vi "Key Event to Bytes.vi"(8 "error in (no error)":errorcluster, 10 "Key Event Data":T1, 11 "Terminal in":refnum<class "Terminal.lvclass">) -> (0 "error out":errorcluster, 2 "String":string, 3 "Terminal out":refnum<class "Terminal.lvclass">)   [LabVIEW 2020, in "Terminal.lvlib" / "Terminal.lvclass"]
uses:
  Terminal.lvclass
  Key Event Data.ctl
  <vilib>/event_ctls.llb/eventvkey.ctl
  Terminal.lvclass/Terminal.ctl
  Terminal.lvlib
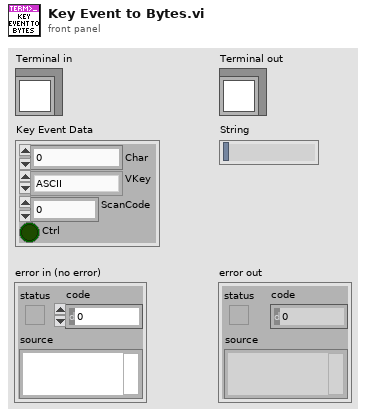
[diagram p1: front panel]
types:
  T1 = typedef "Terminal.lvlib/Key Event Data.ctl" = cluster{"Char":i16, "VKey":T2, "ScanCode":i16, "Ctrl":bool}
  T2 = typedef "eventvkey.ctl" = enum16{"ASCII", "Enter", "Return", "Shift", "Ctrl", "Alt", "Cmd", "Opt", "Caps", "NumLock", "Clear", "Break", "Up", "Down", "Left", "Right", "Insert", "Delete", "Home", "End", "PageUp", "PageDown", "Escape", "Help", "Pause", "ScrollLock", "F1", "F2", "F3", "F4", "F5", "F6", "F7", "F8", "F9", "F10", "F11", "F12", "F13", "F14", "F15", "F16", "F17", "F18", "F19", "F20", "F21", "F22", "F23", "F24", "Play", "VolumeUp", "VolumeDown", "Mute", "Two Byte Char"}
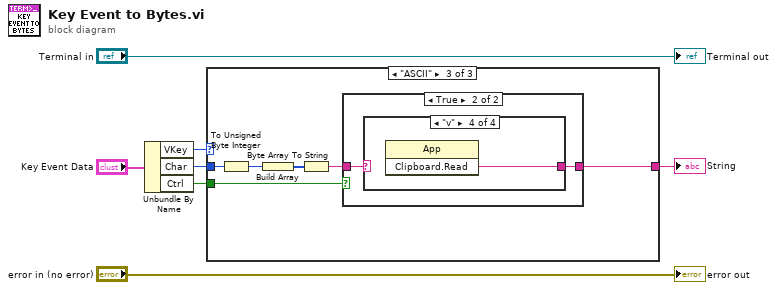
[diagram p0: block diagram]
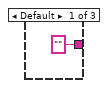
[diagram p2: hidden frame]
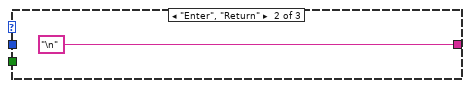
[diagram p3: hidden frame]
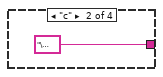
[diagram p6: hidden frame]
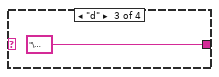
[diagram p7: hidden frame]
diagram:
  n1 = Unbundle By Name("Key Event Data") -> ("VKey"=w3:T2, "Char"=w2:i16, "Ctrl"=w1:bool)
  n2 = case shown="\"ASCII\"" w3 {
    tunnel: w2 -> [_ _ w15]
    tunnel: w1 -> [_ _ w11]
    tunnel: ["" ("Read Clipbrd") "\n" ("Data") w10] -> w5
    frame Default {
    }
    frame "Enter", "Return" {
    }
    frame "ASCII" {
      n3 = To Unsigned Byte Integer(number=w15) -> (unsigned 8bit integer=w14:u8)
      n4 = Build Array(w14) -> (w13:u8[])
      n5 = Byte Array To String(unsigned byte array=w13) -> (string=w12:string)
      n6 = case shown="True" w11 {
        tunnel: w12 -> [w16 w18]
        tunnel: [w16 w17] -> w10
        frame False {
        }
        frame True {
          n7 = case shown="\"v\"" w18 {
            selector: w18 -> [w19 _ _ _]
            tunnel: [w19 "\u0003" ("Data") "\u0004" ("Data") w22] -> w17
            frame Default {
            }
            frame "c" {
            }
            frame "d" {
            }
            frame "v" {
              n8 = invoke class="App" method="Clipboard.Read"() -> ("Read Clipbrd"=w22:string)  [unwired: 3 in, 2 out]
            }
          }
        }
      }
    }
  }
  "String" <- w5
  "error out" <- "error in (no error)"
  "Terminal out" <- "Terminal in"
